vi "time_stamp.vi"(11 "入力ピン":bool) -> (3 "出力値":T1)   [LabVIEW 2023]
uses:
  <vilib>/Utility/miscctls.llb/LVDateTimeRec.ctl
panel:
  in  "曜日表示設定":enum32{"なし", "（月）", "（Mon）", "月曜日"}(tab)
  out "曜日なしの場合の表示":string
  out "（曜日）表示":string
  out "（英語略）表示":string
  out "漢字表示":string
  in  "時間表示設定":T2(tab)
  out "時間と分を表示":string
  out "時間と分と秒を表示":string
  out "時間と分と秒を表示※秒は1/1000秒（ｍS）まで表示":string
  out "時間と分と秒を表示※秒は最小分解能（uS）で表示":string
  out "Get Date/Time Stringパレットを使った時間と分の表示":string
  out "タイムスタンプ値":T3
  # "１秒以下の値"
  # "秒"
  # "分"
  # "時"
  # "日"
  # "月"
  # "年"
  # "曜日表、時間表示の設定は表示したいタブを選択して保存することで設定したことになります。"
  # "曜日を数値化"
  # "今年の１月１日から数えた日数"
  # "サマータイムについての値\n※日本は現在サマータイムがないので０"
  # "."
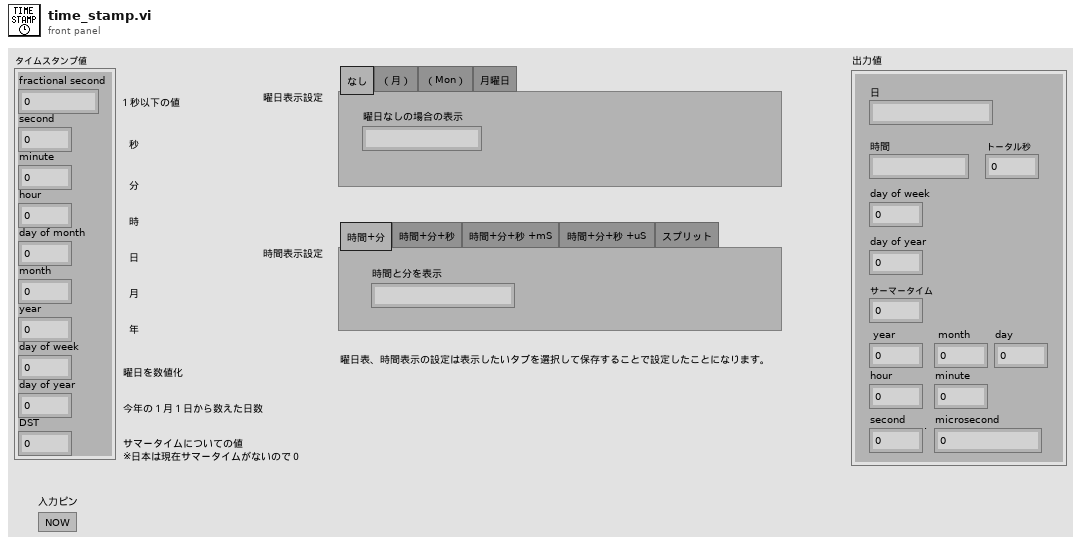
[diagram p1: front panel]
types:
  T1 = cluster{"日":string, "トータル秒":i32, "時間":string, "day of week":i32, "day of year":i32, "サーマータイム":i32, "hour":i32, "minute":i32, "second":i32, "day":i32, " month":i32, " year":i32, "microsecond":i32}
  T2 = enum32{"時間+分", "時間+分+秒", "時間+分+秒 +mS", "時間+分+秒 +uS ", "スプリット"}
  T3 = typedef "LVDateTimeRec.ctl" = cluster{"fractional second":dbl, "second":i32, "minute":i32, "hour":i32, "day of month":i32, "month":i32, "year":i32, "day of week":i32, "day of year":i32, "DST":i32}
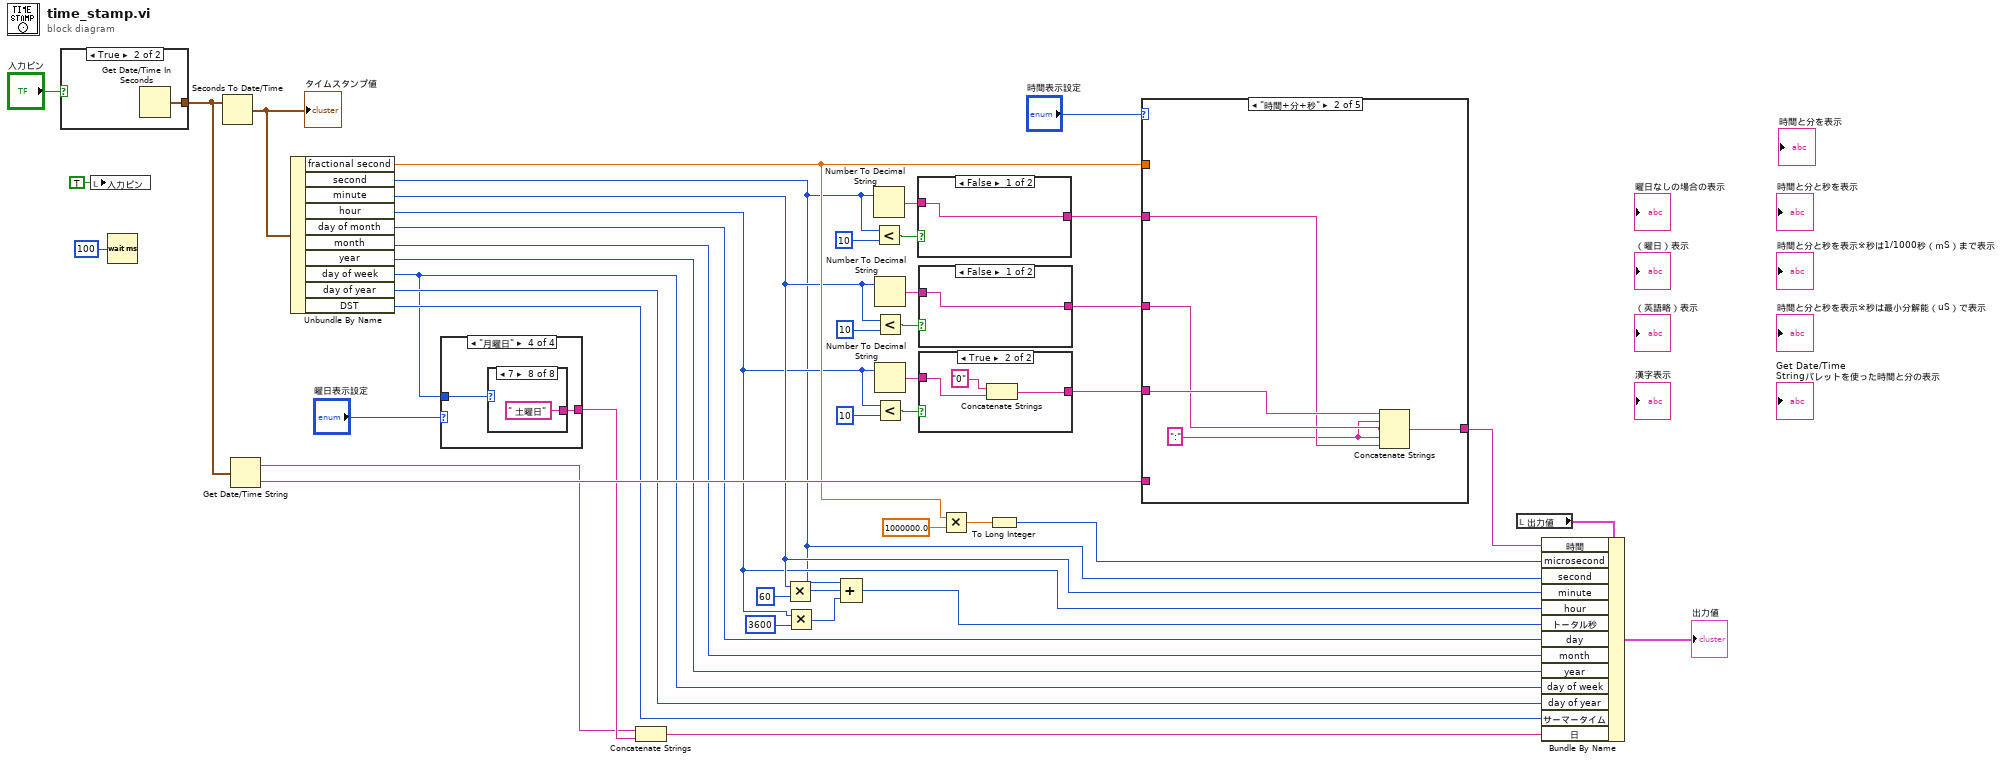
[diagram p0: block diagram]
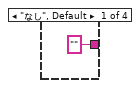
[diagram p2: hidden frame]
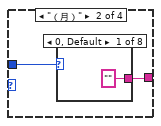
[diagram p3: hidden frame]
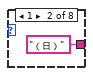
[diagram p4: hidden frame]
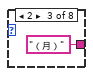
[diagram p5: hidden frame]
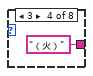
[diagram p6: hidden frame]
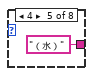
[diagram p7: hidden frame]
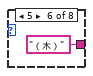
[diagram p8: hidden frame]
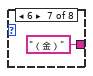
[diagram p9: hidden frame]
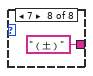
[diagram p10: hidden frame]
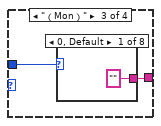
[diagram p11: hidden frame]
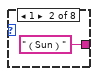
[diagram p12: hidden frame]
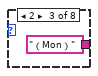
[diagram p13: hidden frame]
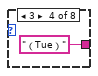
[diagram p14: hidden frame]
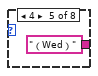
[diagram p15: hidden frame]
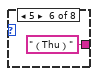
[diagram p16: hidden frame]
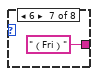
[diagram p17: hidden frame]
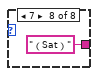
[diagram p18: hidden frame]
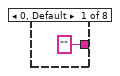
[diagram p19: hidden frame]
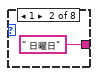
[diagram p20: hidden frame]
diagram:
  n1 = case shown="True" "入力ピン" {
    tunnel: [timestamp(0 s since 1904-01-01) w46] -> w27
    frame False {
    }
    frame True {
      n2 = Get Date/Time In Seconds() -> (seconds since 1Jan1904=w46:timestamp)
    }
  }
  n3 = local write "入力ピン"(TRUE ("Button")) -> ()
  n4 = Wait (ms)(milliseconds to wait=u32 100) -> ()  [unwired: 1 out]
  n5 = Seconds To Date/Time(time stamp (now)=w27) -> (date time rec=w23:T3)  [unwired: 1 in]
  "タイムスタンプ値" <- w23
  n6 = Get Date/Time String(seconds (now)=w27) -> (date string=w20:string, time string=w40:string)  [unwired: 2 in]
  n7 = Unbundle By Name(w23) -> ("fractional second"=w15:dbl, "second"=w1:i32, "minute"=w13:i32, "hour"=w12:i32, "day of month"=w10:i32, "month"=w5:i32, "year"=w4:i32, "day of week"=w6:i32, "day of year"=w7:i32, "DST"=w8:i32)
  n8 = case shown="\"月曜日\"" "曜日表示設定" {
    tunnel: ["" w48 w58 w68] -> w21
    tunnel: w6 -> [_ w49 w59 w69]
    frame "なし", Default {
    }
    frame "（月）" {
      n9 = case shown="0, Default" w49 {
        tunnel: ["" "（日）" "（月）" "（火）" "（水）" "（木）" "（金）" "（土）"] -> w48
        frame 0, Default {
        }
        frame 1 {
        }
        frame 2 {
        }
        frame 3 {
        }
        frame 4 {
        }
        frame 5 {
        }
        frame 6 {
        }
        frame 7 {
        }
      }
    }
    frame "（Mon）" {
      n10 = case shown="0, Default" w59 {
        tunnel: ["" "（Sun）" "（Mon）" "（Tue）" "（Wed）" "（Thu）" "（Fri）" "（Sat）"] -> w58
        frame 0, Default {
        }
        frame 1 {
        }
        frame 2 {
        }
        frame 3 {
        }
        frame 4 {
        }
        frame 5 {
        }
        frame 6 {
        }
        frame 7 {
        }
      }
    }
    frame "月曜日" {
      n11 = case shown="7" w69 {
        tunnel: ["" " 日曜日" " 月曜日" " 火曜日" " 水曜日" " 木曜日" " 金曜日" " 土曜日"] -> w68
        frame 0, Default {
        }
        frame 1 {
        }
        frame 2 {
        }
        frame 3 {
        }
        frame 4 {
        }
        frame 5 {
        }
        frame 6 {
        }
        frame 7 {
        }
      }
    }
  }
  n12 = Concatenate Strings(w20, w21) -> (w9:string)
  n13 = Multiply(x=w13, y=60) -> (x*y=w42:i32)
  n14 = Multiply(x=w12, y=3600) -> (x*y=w41:i32)
  n15 = Compound Arithmetic op=ADD(w1, w42, w41) -> (w11:i32)
  n16 = Number To Decimal String(number=w1) -> (decimal integer string=w38:string)  [unwired: 1 in]
  n17 = Less?(x=w1, y=10) -> (x < y?=w39:bool)
  n18 = Number To Decimal String(number=w13) -> (decimal integer string=w34:string)  [unwired: 1 in]
  n19 = Less?(x=w13, y=10) -> (x < y?=w35:bool)
  n20 = Number To Decimal String(number=w12) -> (decimal integer string=w31:string)  [unwired: 1 in]
  n21 = Less?(x=w12, y=10) -> (x < y?=w32:bool)
  n22 = case shown="False" w39 {
    tunnel: w38 -> [w78 w81]
    tunnel: [w78 w80] -> w36
    frame False {
    }
    frame True {
      n23 = Concatenate Strings("0" ("string"), w81) -> (w80:string)
    }
  }
  n24 = case shown="False" w35 {
    tunnel: w34 -> [w82 w85]
    tunnel: [w82 w84] -> w28
    frame False {
    }
    frame True {
      n25 = Concatenate Strings("0" ("string"), w85) -> (w84:string)
    }
  }
  n26 = case shown="True" w32 {
    tunnel: w31 -> [w86 w89]
    tunnel: [w86 w88] -> w29
    frame False {
    }
    frame True {
      n27 = Concatenate Strings("0" ("string"), w89) -> (w88:string)
    }
  }
  n28 = Multiply(x=w15, y=1000000.0) -> (x*y=w14:dbl)
  n29 = To Long Integer(number=w14) -> (32bit integer=w2:i32)
  n30 = case shown="\"時間+分+秒\"" "時間表示設定" {
    tunnel: w36 -> [_ w95 w108 w118 _]
    tunnel: w28 -> [w91 w97 w109 w119 _]
    tunnel: w29 -> [w90 w98 w110 w120 _]
    tunnel: [w92 w96 w106 w116 w122] -> w3
    tunnel: w15 -> [_ _ w102 w112 _]
    tunnel: w40 -> [_ _ _ _ w122]
    frame "時間+分", Default {
      n31 = Concatenate Strings(w90, ":" ("string"), w91) -> (w92:string)
    }
    frame "時間+分+秒" {
      w94 = ":" ("string")
      n32 = Concatenate Strings(w98, w94, w97, w94, w95) -> (w96:string)
    }
    frame "時間+分+秒 +mS" {
      w107 = ":" ("string")
      n33 = Multiply(x=w102, y=1000.0) -> (x*y=w105:dbl)
      n34 = Round To Nearest(number=w105) -> (nearest integer value=w103:dbl)
      n35 = To Long Integer(number=w103) -> (32bit integer=w99:i32)
      n36 = Number To Decimal String(number=w99) -> (decimal integer string=w100:string)  [unwired: 1 in]
      n37 = Concatenate Strings(w110, w107, w109, w107, w108, "." ("string"), w100) -> (w106:string)
    }
    frame "時間+分+秒 +uS " {
      w121 = ":" ("string")
      n38 = Multiply(x=w112, y=1000000.0) -> (x*y=w113:dbl)
      n39 = To Long Integer(number=w113) -> (32bit integer=w114:i32)
      n40 = Number To Decimal String(number=w114) -> (decimal integer string=w115:string)  [unwired: 1 in]
      n41 = Concatenate Strings(w120, w121, w119, w121, w118, "." ("string"), w115) -> (w116:string)
    }
    frame "スプリット" {
    }
  }
  n42 = local read "出力値"() -> (w18:T1)
  n43 = Bundle By Name(cluster=w18, "時間"=w3, "microsecond"=w2, "second"=w1, "minute"=w13, "hour"=w12, "トータル秒"=w11, "day"=w10, "month"=w5, "year"=w4, "day of week"=w6, "day of year"=w7, "サーマータイム"=w8, "日"=w9) -> (→"出力値":T1)
